vi "labview.vi"() -> ()   [LabVIEW 2022 SP3]
uses:
  <vilib>/MakerHub/LINX/Public/Peripherals/Analog/Analog Read 1 Chan.vi
  <vilib>/MakerHub/LINX/Public/Peripherals/PWM/PWM Set Duty Cycle 1 Chan.vi
  <vilib>/MakerHub/LINX/Public/Peripherals/Digital/Digital Read 1 Chan.vi
  <vilib>/MakerHub/LINX/Public/Peripherals/Digital/Digital Write 1 Chan.vi
  <vilib>/MakerHub/LINX/Public/Peripherals/Analog/Analog Read N Chans.vi
  <vilib>/MakerHub/LINX/Public/Peripherals/Digital/Digital Read N Chans.vi
  <vilib>/MakerHub/LINX/Public/Peripherals/Digital/Digital Write N Chans.vi
  <vilib>/MakerHub/LINX/Private/Local IO/LinxAnalogRead.vi
  <vilib>/MakerHub/LINX/Public/Utilities/Check Channel.vi
  <vilib>/MakerHub/LINX/Private/Local IO/LinxDigitalRead.vi
  <vilib>/MakerHub/LINX/Private/Local IO/LinxDigitalWrite.vi
  <vilib>/MakerHub/LINX/Public/Utilities/Open Serial.vi
  <vilib>/MakerHub/LINX/Public/Sensors/Motion/Servo/Servo Open One Channel.vi
  <vilib>/MakerHub/LINX/Private/Utilties/Generate Error.vi
  <vilib>/MakerHub/LINX/Public/Peripherals/PWM/PWM Set Duty Cycle N Chans.vi
  <vilib>/MakerHub/LINX/Public/Sensors/Motion/Servo/Servo Set Pulse Width One Channel.vi
  <vilib>/MakerHub/LINX/Public/Sensors/Motion/Servo/Servo Close One Channel.vi
  <vilib>/MakerHub/LINX/LMH-LINX.lvlib
  <vilib>/MakerHub/LINX/Public/Sensors/Motion/Servo/Servo.lvlib
panel:
  out "BUZZER":bool
  out "FAN":bool
  out "YELLOW light":bool
  out "GREEN light":bool
  out "RED light":bool
  out "analoge A0 LDR":dbl
  out "analog A4 LDR":dbl
  out "Thermometer":dbl(slide) scale=0.0..100.0
  in  "stop":bool
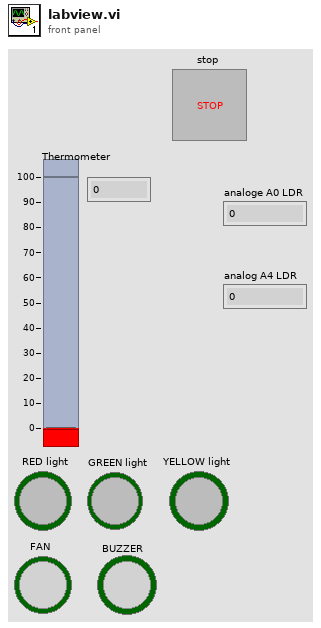
[diagram p1: front panel]
types:
  T1 = typedef "LMH-LINX.lvlib/LINX Ref.ctl" = cluster{"IO":T2, "Interface":T3, "LINX Device Config":T4}
  T2 = typedef "LMH-LINX.lvlib/Platform.ctl" = enum16{"Remote", "Local"}
  T3 = typedef "LMH-LINX.lvlib/Interface.ctl" = enum16{"Serial", "TCP"}
  T4 = typedef "LMH-LINX.lvlib/Device.lvlib/LINX Device Config.ctl" = cluster{"Interface":T3, "COM Port":refnum<visa-resource-name>, "TCP Configuration":T5, "Device Family":u8, "Device ID":u8, "Device Name":string, "TCP Ref":refnum<k5>, "Channels":T6}
  T5 = typedef "LMH-LINX.lvlib/Device.lvlib/TCP Config.ctl" = cluster{"IP Address":string, "Port":u16}
  T6 = typedef "LMH-LINX.lvlib/Channels.ctl" = cluster{"DI":u8[], "DO":u8[], "AI":u8[], "AO":u8[], "PWM":u8[], "QE":u8[], "UART":u8[], "I2C 2":u8[], "SPI":u8[], "CAN":u8[], "Servo":u8[], "AI Ref (V)":dbl, "AI Resolution (Bits)":u8, "AO Ref (V)":dbl, "AO Resolution (Bits)":u8}
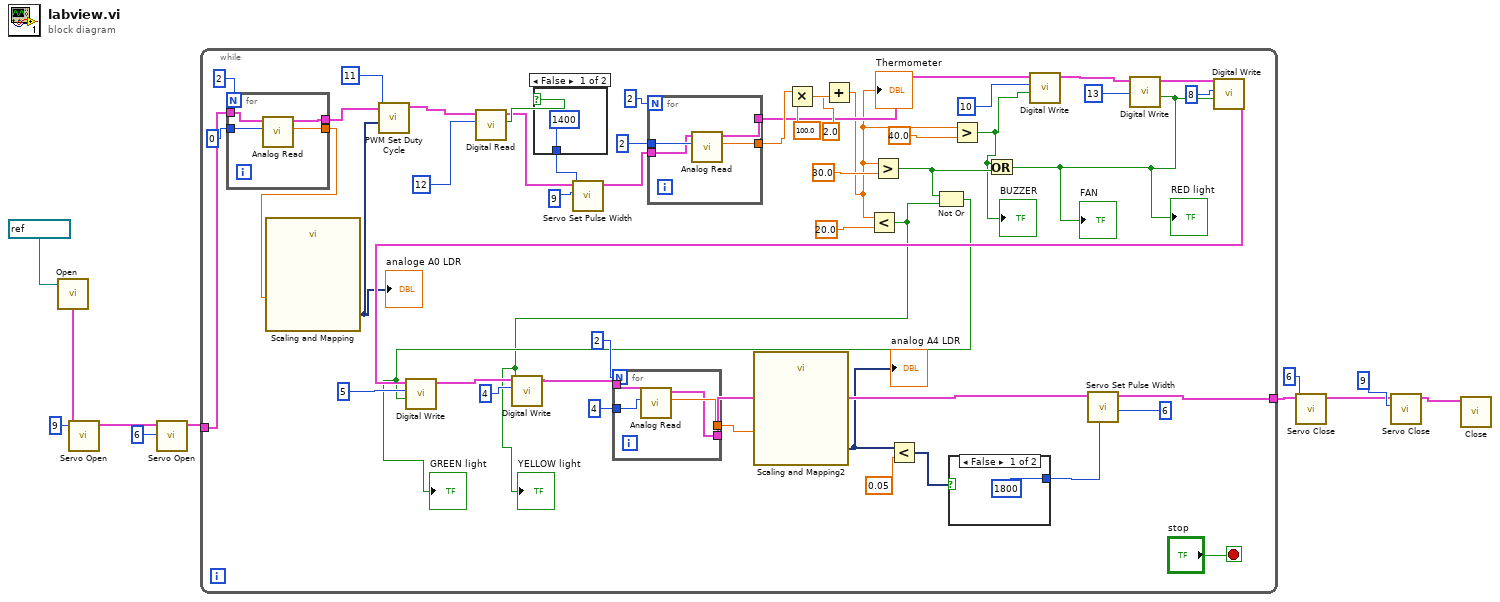
[diagram p0: block diagram]
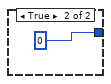
[diagram p2: hidden frame]
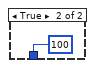
[diagram p3: hidden frame]
diagram:
  n1 = call-poly <vilib>:"Open.vi"("Serial Port"=refnum<visa-resource-name> "COM3") -> ("LINX Resource"=w10:T1)  [unwired: 8 in, 2 out]
  n2 = call-poly <vilib>:"Servo Open.vi"("Servo Channel"=u8 9, "LINX Resource"=w10) -> ("LINX Resource"=w6:T1)  [unwired: 8 in, 1 out]
  n3 = call-poly <vilib>:"Servo Open.vi"("Servo Channel"=u8 6, "LINX Resource"=w6) -> ("LINX Resource"=w5:T1)  [unwired: 8 in, 1 out]
  n4 = while {
    tunnel: [w28] -> w3
    tunnel: w5 -> [w40]
    stop <- "stop" stop-if-true
    n5 = for {
      N: 2 -> [_]
      tunnel: u8 0 ("Analog Channel") -> [w76]
      tunnel: w40 -> [w75]
      tunnel: [w74] -> w39
      tunnel: [w73] -> w38
      n6 = call-poly <vilib>:"Analog Read.vi"("Analog Channel"=w76, "LINX Resource"=w75) -> ("Voltage"=w74:dbl, "LINX Resource"=w73:T1)  [unwired: 6 in, 2 out]
    }
    n7 = call "Scaling and Mapping"("Signals"=w39) -> ("Scaled Signals"=w17:dynamicdata)  [unwired: 9 in, 1 out]
    "analoge A0 LDR" <- w17
    n8 = call-poly <vilib>:"PWM Set Duty Cycle.vi"("Duty Cycle (0-1)"=w17, "PWM Channel"=u8 11, "LINX Resource"=w38) -> ("LINX Resource"=w48:T1)  [unwired: 7 in, 1 out]
    n9 = call-poly <vilib>:"Digital Read.vi"("DI Channel"=u8 12, "LINX Resource"=w48) -> ("DI Value"=w58:bool, "LINX Resource"=w47:T1)  [unwired: 7 in, 1 out]
    n10 = case shown="False" w58 {
      tunnel: [1400 100] -> w61
      frame False {
      }
      frame True {
      }
    }
    n11 = call-poly <vilib>:"Servo Set Pulse Width.vi"("Pulse Width (uS)"=w61, "Servo Channel"=u8 9, "LINX Resource"=w47) -> ("LINX Resource"=w35:T1)  [unwired: 7 in, 1 out]
    n12 = for {
      N: 2 -> [_]
      tunnel: u8 2 ("Analog Channel") -> [w72]
      tunnel: w35 -> [w71]
      tunnel: [w70] -> w34
      tunnel: [w69] -> w33
      n13 = call-poly <vilib>:"Analog Read.vi"("Analog Channel"=w72, "LINX Resource"=w71) -> ("Voltage"=w70:dbl, "LINX Resource"=w69:T1)  [unwired: 6 in, 2 out]
    }
    n14 = Multiply(x=w34, y=100.0) -> (x*y=w55:dbl)
    n15 = Add(x=w55, y=2.0) -> (x+y=w12:dbl)
    "Thermometer" <- w12
    n16 = Less?(x=w12, y=20.0) -> (x < y?=w15:bool)
    "YELLOW light" <- w15
    n17 = Greater?(x=w12, y=30.0 ("x")) -> (0:w29:bool)
    n18 = Not Or(1:w15, 2:w29) -> (0:w16:bool)
    "GREEN light" <- w16
    n19 = Greater?(x=w12, y=40.0) -> (0:w13:bool)
    "BUZZER" <- w13
    n20 = Or(x=w13, y=w29) -> (x .or. y?=w14:bool)
    "RED light" <- w14
    "FAN" <- w14
    n21 = call-poly <vilib>:"Digital Write.vi"("Output Value"=w13, "DO Channel"=u8 10, "LINX Resource"=w33) -> ("LINX Resource"=w46:T1)  [unwired: 7 in, 1 out]
    n22 = call-poly <vilib>:"Digital Write.vi"("Output Value"=w14, "DO Channel"=u8 13, "LINX Resource"=w46) -> ("LINX Resource"=w45:T1)  [unwired: 7 in, 1 out]
    n23 = call-poly <vilib>:"Digital Write.vi"("Output Value"=w14, "DO Channel"=u8 8, "LINX Resource"=w45) -> ("LINX Resource"=w44:T1)  [unwired: 7 in, 1 out]
    n24 = call-poly <vilib>:"Digital Write.vi"("Output Value"=w16, "DO Channel"=u8 5, "LINX Resource"=w44) -> ("LINX Resource"=w43:T1)  [unwired: 7 in, 1 out]
    n25 = call-poly <vilib>:"Digital Write.vi"("Output Value"=w15, "DO Channel"=u8 4, "LINX Resource"=w43) -> ("LINX Resource"=w25:T1)  [unwired: 7 in, 1 out]
    n26 = for {
      N: 2 -> [_]
      tunnel: u8 4 ("Analog Channel") -> [w66]
      tunnel: w25 -> [w65]
      tunnel: [w64] -> w24
      tunnel: [w63] -> w23
      n27 = call-poly <vilib>:"Analog Read.vi"("Analog Channel"=w66, "LINX Resource"=w65) -> ("Voltage"=w64:dbl, "LINX Resource"=w63:T1)  [unwired: 6 in, 2 out]
    }
    n28 = call "Scaling and Mapping2"("Signals"=w24) -> ("Scaled Signals"=w18:dynamicdata)  [unwired: 9 in, 1 out]
    "analog A4 LDR" <- w18
    n29 = Less?(x=w18, y=0.05) -> (x < y?=w20:dynamicdata)
    n30 = case shown="False" w20 {
      tunnel: [1800 0] -> w19
      frame False {
      }
      frame True {
      }
    }
    n31 = call-poly <vilib>:"Servo Set Pulse Width.vi"("Pulse Width (uS)"=w19, "Servo Channel"=u8 6, "LINX Resource"=w23) -> ("LINX Resource"=w28:T1)  [unwired: 7 in, 1 out]
  }
  n32 = call-poly <vilib>:"Servo Close.vi"("Servo Channel"=u8 6, "LINX Resource"=w3) -> ("LINX Resource"=w2:T1)  [unwired: 8 in, 1 out]
  n33 = call-poly <vilib>:"Servo Close.vi"("Servo Channel"=u8 9, "LINX Resource"=w2) -> ("LINX Resource"=w11:T1)  [unwired: 8 in, 1 out]
  n34 = call <vilib>:"Close.vi"("LINX Resource"=w11) -> ()  [unwired: 10 in, 1 out]
